vi "Create DVR.vi"(11 "Error In":errorcluster) -> (4 "message type classes":string[](array[string]), 6 "Type DVR Ref":T2[](array[typedef]), 8 "Message data classes":string[](array[string]), 10 "Data DVR Ref":T1[](array[typedef]), 15 "Error Out":errorcluster)   [LabVIEW 2023, in "Message Type.lvclass"]
uses:
  Message Type.lvclass
  Controls/Type Class Ref.ctl
  Controls/Class DVR Ref.ctl
  Message Data/Message Data.lvclass
  Message Type.lvclass/Message Type.ctl
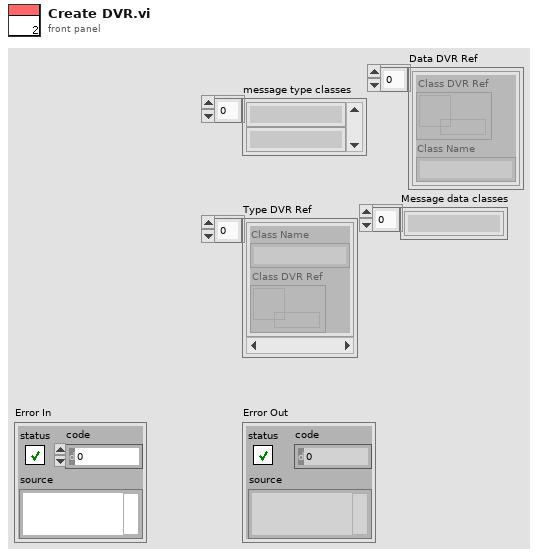
[diagram p1: front panel]
types:
  T1 = typedef "Class DVR Ref.ctl" = cluster{"Class DVR Ref":refnum<data-value>, "Class Name":string}
  T2 = typedef "Type Class Ref.ctl" = cluster{"Class Name":string, "Class DVR Ref":refnum<data-value>}
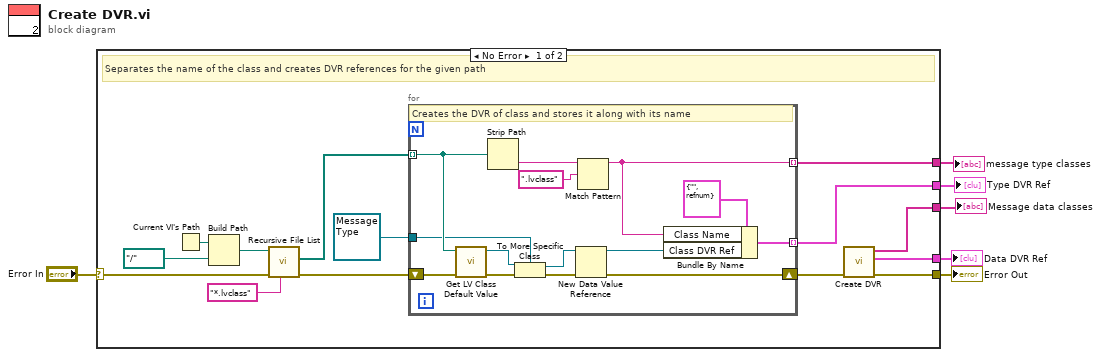
[diagram p0: block diagram]
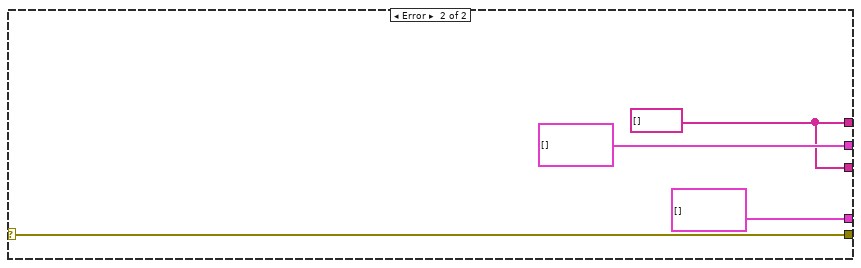
[diagram p2: hidden frame]
diagram:
  n1 = case shown="No Error" "Error In" {
    selector: "Error In" -> [w13 w38]
    tunnel: [w9 w38] -> w5
    tunnel: [w18 w36] -> w4
    tunnel: [w10 T2[] []] -> w3
    tunnel: [w8 w36] -> w1
    tunnel: [w7 T1[] [] ("DVR Ref")] -> w2
    frame No Error {
      # "Separates the name of the class and creates DVR references for the given path"
      n2 = Current VI's Path() -> (path=w16:path)
      n3 = Build Path(base path=w16, name or relative path=path "../..") -> (appended path=w15:path)
      n4 = call <vilib>:"Recursive File List.vi"("pattern"="*.lvclass", "error in (no error)"=w13, "Folder Path"=w15) -> ("error out"=w12:errorcluster, "All Files in Dir"=w11:path[])  [unwired: 4 in, 3 out]
      n5 = for {
        tunnel: w11 -> [w31] mode=indexing
        tunnel: [w21] -> w18 mode=indexing
        shift-right: [w27] -> w19
        shift-left: w12 -> [w33]
        tunnel: refnum<class "Message Type.lvclass"> refnum ("Arithemetic Operation in") -> [w30]
        tunnel: [w24] -> w10 mode=indexing
        # "Creates the DVR of class and stores it along with its name"
        n6 = call <vilib>:"Get LV Class Default Value.vi"("error in (no error)"=w33, "class path"=w31) -> ("error out"=w32:errorcluster, "object"=w29:refnum<class>)  [unwired: 8 in]
        n7 = Strip Path(path=w31) -> (name=w25:string)  [unwired: 1 out]
        n8 = To More Specific Class(target class=w30, reference=w29, error in=w32) -> (specific class reference=w26:refnum<class "Message Type.lvclass">, error out=w28:errorcluster)
        n9 = New Data Value Reference(data value=w26, error in=w28) -> (data value reference=w22:refnum<data-value>, error out=w27:errorcluster)
        n10 = Match Pattern(string=w25, regular expression=".lvclass") -> (before substring=w21:string)  [unwired: 1 in, 3 out]
        n11 = Bundle By Name(cluster=T2 {"Class Name"="", "Class DVR Ref"=refnum} ("Type Class"), "Class Name"=w21, "Class DVR Ref"=w22) -> (w24:T2)
      }
      n12 = call "Create DVR.vi"("Error In"=w19) -> ("Error Out"=w9:errorcluster, "DVR Ref"=w7:T1[], "Class Names"=w8:string[])  [unwired: 8 in]
    }
    frame Error {
      w36 = string[] []
    }
  }
  "Error Out" <- w5
  "Type DVR Ref" <- w3
  "message type classes" <- w4
  "Data DVR Ref" <- w2
  "Message data classes" <- w1
